vi "Read TempSP.vi"(8 "error in (no error)":errorcluster, 11 "ThermPID in":refnum<class "ThermPID.lvclass">) -> (0 "error out":errorcluster, 2 "SetPoint (C)":dbl, 3 "ThermPID out":refnum<class "ThermPID.lvclass">)   [LabVIEW 2023, in "ThermPID.lvclass"]
uses:
  ThermPID.lvclass
  ThermPID.lvclass/ThermPID.ctl
  PIDController/PIDController.lvclass
  <vilib>/NI/Modbus Library/API/Master/Modbus Master.lvclass
  PIDModBus/Controls/Register Enum.ctl
  PIDModBus/PIDModbus.lvlib
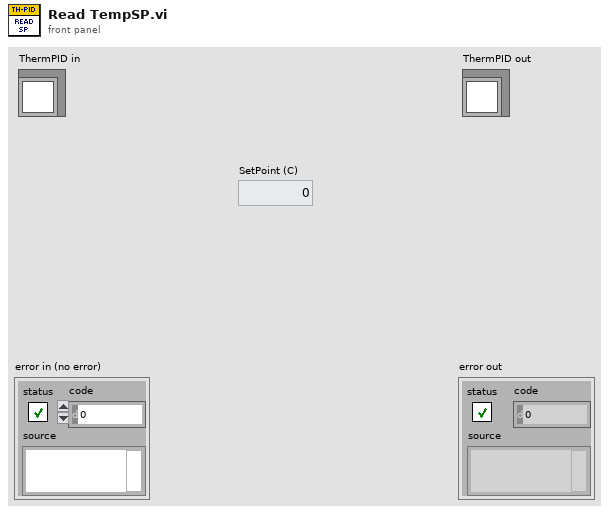
[diagram p1: front panel]
types:
  T1 = typedef "PIDModbus.lvlib/Register Enum.ctl" = u16
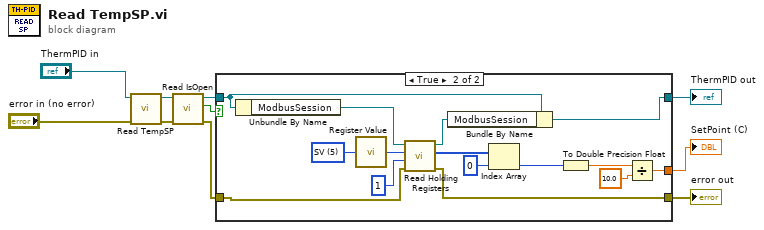
[diagram p0: block diagram]
diagram:
  n1 = call-parent "Read TempSP.vi"("error in (no error)"="error in (no error)", "PIDController in"="ThermPID in") -> ("error out"=w3:errorcluster, "PIDController out"=w8:refnum<class "ThermPID.lvclass">)  [unwired: 7 in, 1 out]
  n2 = call-dynamic "Read IsOpen.vi"("error in (no error)"=w3, "PIDController in"=w8) -> ("error out"=w2:errorcluster, "IsOpen"=w1:bool, "PIDController out"=w7:refnum<class "ThermPID.lvclass">)  [unwired: 7 in]
  n3 = case shown="True" w1 {
    tunnel: w7 -> [w12 w18]
    tunnel: [w12 w17] -> w6
    tunnel: [w11 w15] -> w5
    tunnel: [_ w14] -> w4
    tunnel: w2 -> [w11 w13]
    frame False {
    }
    frame True {
      w25 = T1 5 items=["PV"=0, "SV"=5, "P1"=24, "I1"=25, "D1"=26] ("Register")
      n4 = Unbundle By Name(w18) -> ("ModbusSession"=w19:refnum<class "Modbus Master.lvclass">)
      n5 = call "Register Value.vi"("Register"=w25) -> ("RegAddr (Hex)"=w24:u16)
      n6 = call-dynamic "Read Holding Registers.vi"("error in"=w13, "number of inputs"=u16 1, "starting address"=w24, "Modbus master in"=w19) -> ("error out"=w15:errorcluster, "register values"=w27:u16[], "Modbus master out"=w16:refnum<class "Modbus Master.lvclass">)  [unwired: 5 in]
      n7 = Bundle By Name(cluster=w18, "ModbusSession"=w16) -> (w17:refnum<class "ThermPID.lvclass">)
      n8 = Index Array(array=w27, index=0) -> (element=w22:u16)
      n9 = To Double Precision Float(number=w22) -> (double precision float=w20:dbl)
      n10 = Divide(x=w20, y=10.0) -> (x/y=w14:dbl)
    }
  }
  "error out" <- w5
  "ThermPID out" <- w6
  "SetPoint (C)" <- w4
